vi "Read Timeout.vi"(8 "error in (no error)":errorcluster, 11 "REST Client in":refnum<class "REST Client.lvclass">) -> (0 "error out":errorcluster, 2 "Timeout":i32, 3 "REST Client out":refnum<class "REST Client.lvclass">)   [LabVIEW 2018, in "REST Client_JKI.lvlib" / "REST Client.lvclass"]
doc: "Read Timeout value"
uses:
  REST Client.lvclass
  REST Client.lvclass/REST Client.ctl
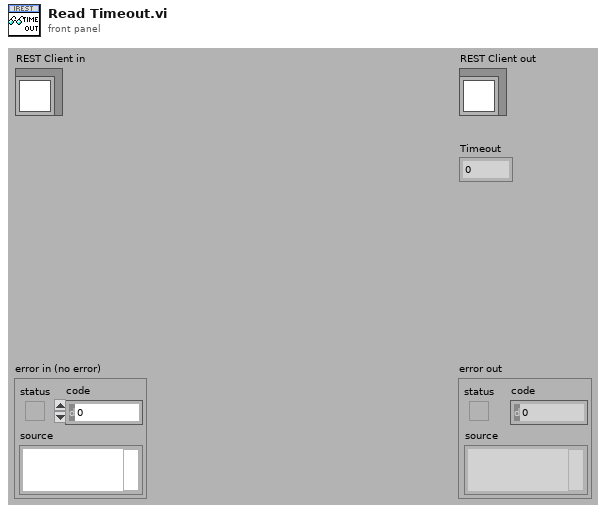
[diagram p1: front panel]
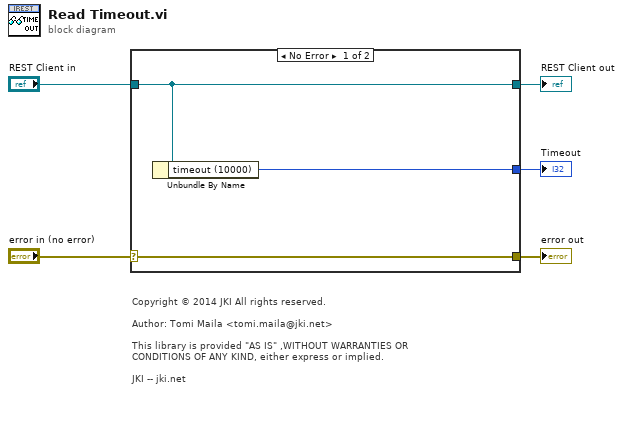
[diagram p0: block diagram]
diagram:
  # "Copyright © 2014 JKI All rights reserved.\n\nAuthor: Tomi Maila <tomi.maila@jki.net>\n\nThis library is provided \"AS IS\" ,WITHOUT WARRANTIES OR \nCONDITIONS OF ANY KIND, either express or implied.\n\nJKI -- jki.net"
  n1 = case shown="No Error" "error in (no error)" {
    selector: "error in (no error)" -> [w8 w9]
    tunnel: [w8 w9] -> w4
    tunnel: [w7 w10] -> w2
    tunnel: "REST Client in" -> [w7 w10]
    tunnel: [w6 _] -> w1
    frame No Error {
      n2 = Unbundle By Name(w7) -> ("timeout (10000)"=w6:i32)
    }
    frame Error {
    }
  }
  "error out" <- w4
  "REST Client out" <- w2
  "Timeout" <- w1
